vi "Impedance tube v0.3_cross_power.vi"() -> ()   [LabVIEW 2021]
uses:
  <vilib>/Analysis/2dsp.llb/Real FFT.vi
  <vilib>/express/express arith-compare/Formula/XNode/ExpressFormulaBlockNode.xnode
  <vilib>/Analysis/NI_AALPro.lvlib
panel:
  out "Transfer function 2":dbl[](graph)
  in  "dt":dbl=1.0 format="%0.2f"
  out "probe 1":dbl[](graph)
  out "Reflection coefficient":dbl[](graph)
  out "Absorption Coefficient":dbl[](graph)
  out "FFT {2}":cdb[](array[numeric])
  out "FFT {1}":cdb[](array[numeric])
  out "Transfer function":dbl[](graph)
  out "MIC 2":dynamicdata(graph)
  out "FFT2":dbl[](graph)
  in  "FFT size 2":i32=-1
  out "MIC 2":dbl
  out "FFT1":dbl[](graph)
  out "MIC 1":dynamicdata(graph)
  in  "FFT size":i32=-1
  out "MIC 1":dbl
  in  "stop (F)":bool
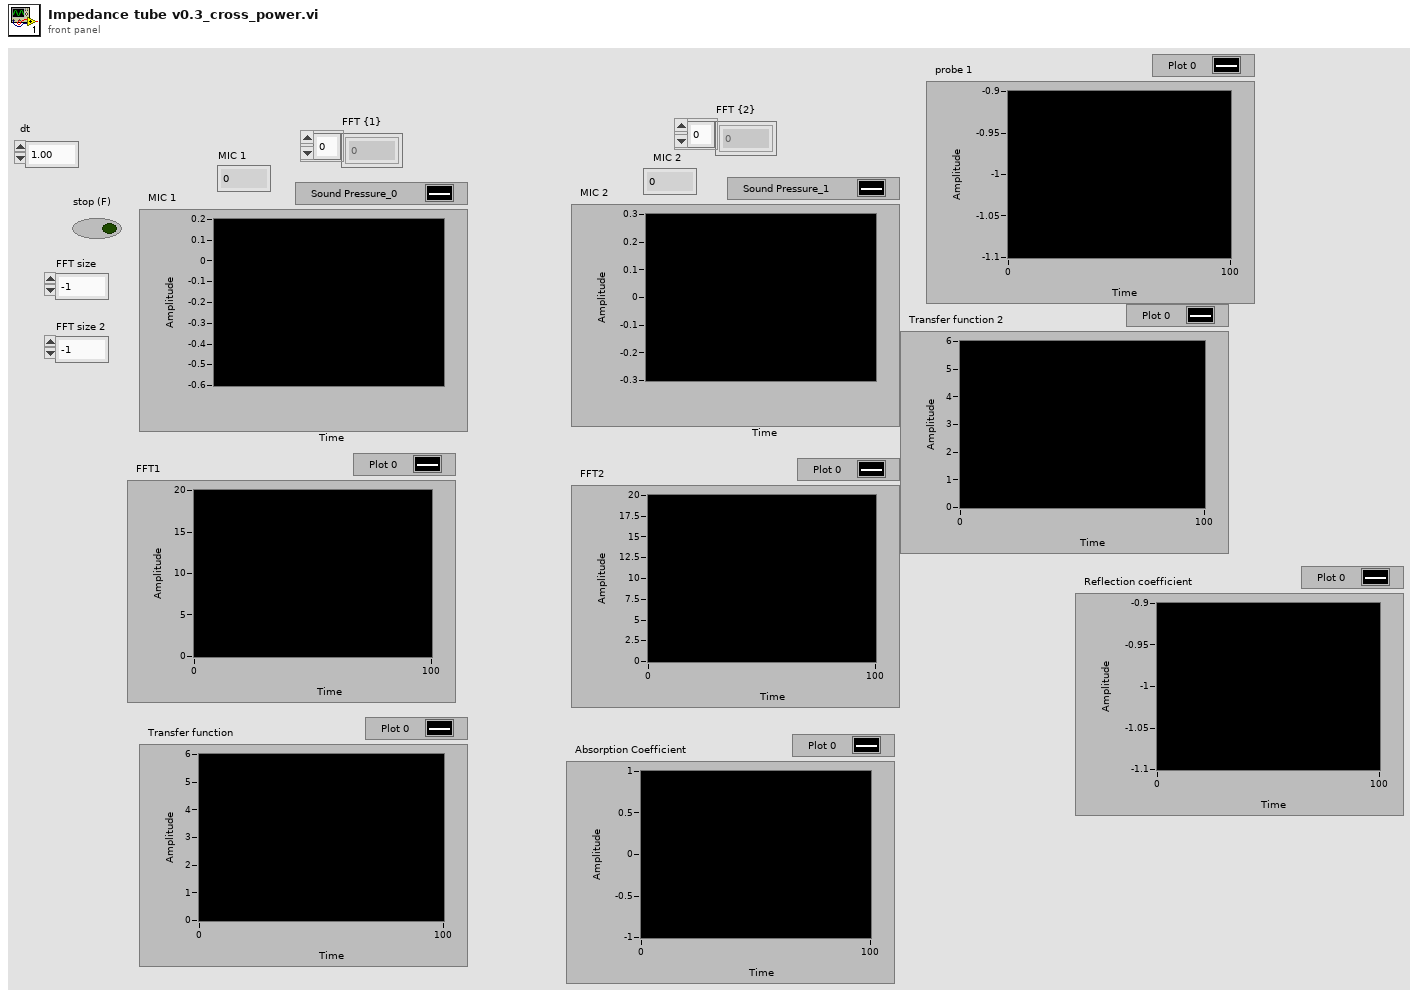
[diagram p1: front panel]
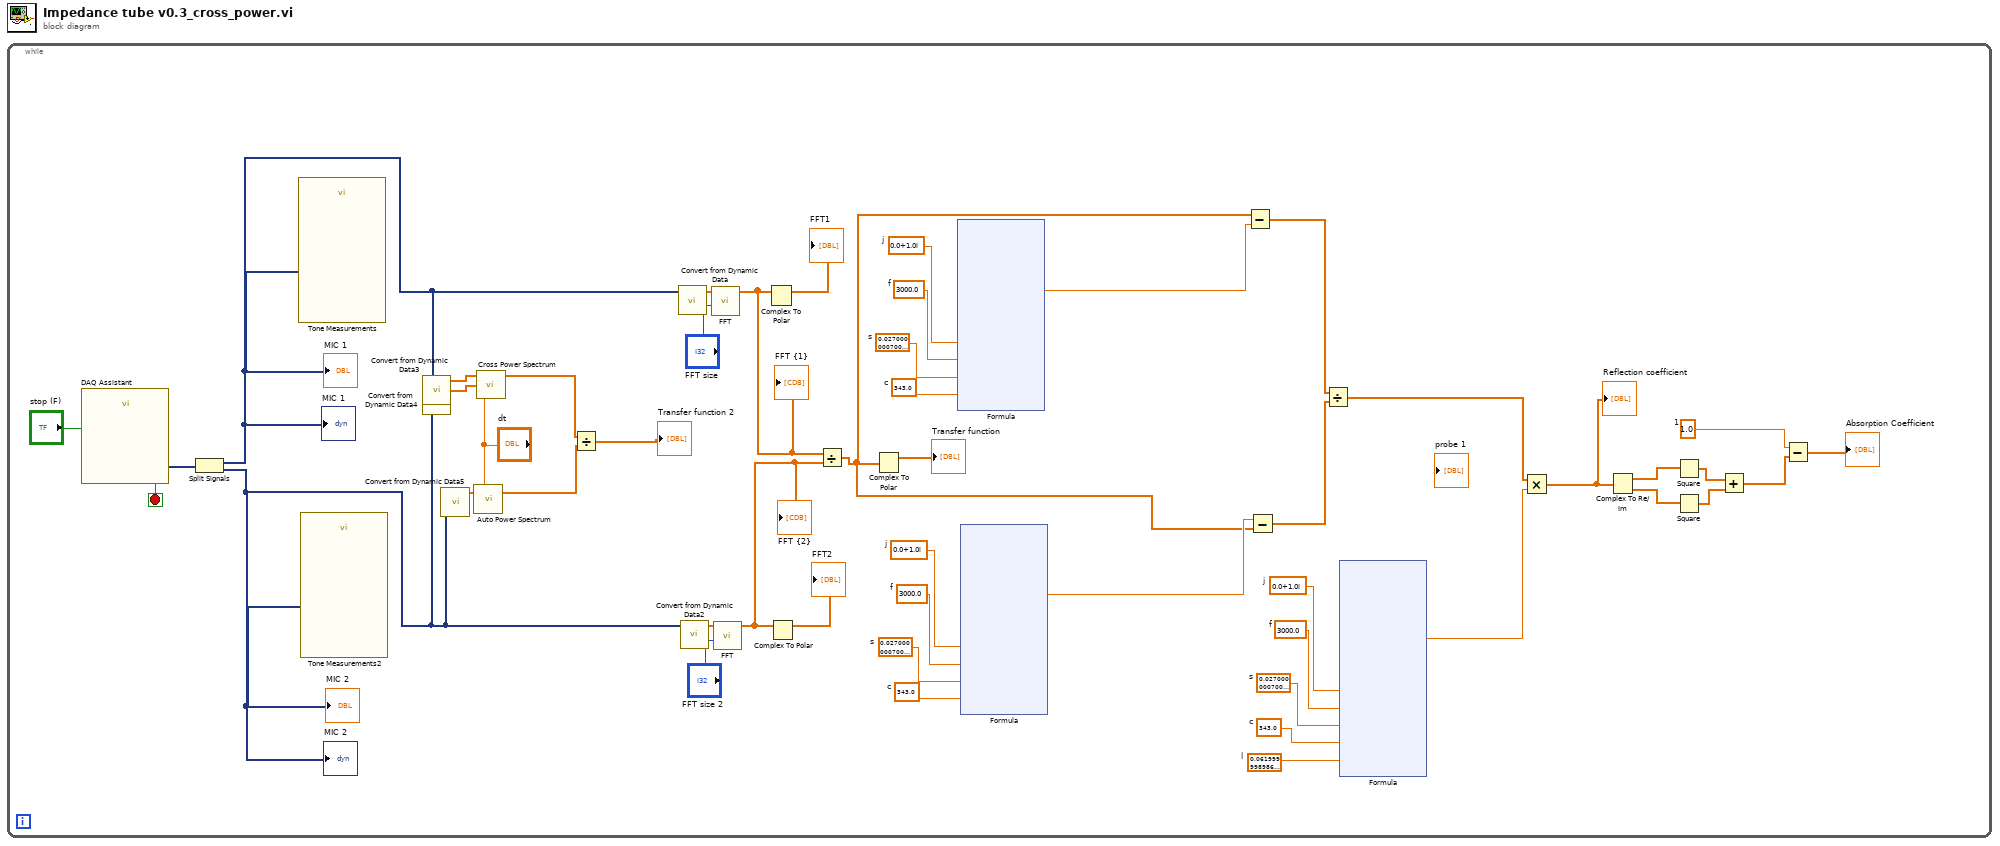
[diagram p0: block diagram]
diagram:
  n1 = while {
    stop <- w48 stop-if-true
    w17 = sgl 1.0  # 1
    w23 = sgl 0.062  # l
    w26 = sgl 3000.0  # f
    w25 = sgl 0.027  # s
    w24 = sgl 343.0  # c
    w27 = csg 0.0+1.0i  # j
    w31 = sgl 3000.0  # f
    w30 = sgl 0.027  # s
    w29 = sgl 343.0  # c
    w32 = csg 0.0+1.0i  # j
    w36 = sgl 3000.0  # f
    w35 = sgl 0.027  # s
    w34 = sgl 343.0  # c
    w37 = csg 0.0+1.0i  # j
    n2 = call "DAQ Assistant"("stop (F)"="stop (F)") -> ("data"=w44:dynamicdata, "stopped"=w48:bool)  [unwired: 15 in, 2 out]
    n3 = Split Signals(w44) -> (w9:dynamicdata, w6:dynamicdata)  [unwired: 2 in]
    "MIC 1" <- w9
    "MIC 1" <- w9
    "MIC 2" <- w6
    "MIC 2" <- w6
    n4 = call "Tone Measurements"("Signals"=w9) -> ()  [unwired: 8 in, 3 out]
    n5 = call "Tone Measurements2"("Signals"=w6) -> ()  [unwired: 8 in, 3 out]
    n6 = call "Convert from Dynamic Data3"("Dynamic Data Type"=w9) -> ("Array"=w8:dbl[])  [unwired: 3 in]
    n7 = call "Convert from Dynamic Data4"("Dynamic Data Type"=w6) -> ("Array"=w7:dbl[])  [unwired: 3 in]
    n8 = call "Convert from Dynamic Data5"("Dynamic Data Type"=w6) -> ("Array"=w5:dbl[])  [unwired: 3 in]
    n9 = call <vilib>:"Auto Power Spectrum.vi"("dt"="dt", "Signal (V)"=w5) -> ("Power Spectrum (V^2 rms)"=w2:dbl[])  [unwired: 1 out]
    n10 = call <vilib>:"Cross Power Spectrum.vi"("dt"="dt", "Signal Y (V)"=w7, "Signal X (V)"=w8) -> ("Cross Power XY Spectrum Mag (V^2rms)"=w3:dbl[])  [unwired: 2 out]
    n11 = Divide(x=w3, y=w2) -> (x/y=→"Transfer function 2":dbl[])
    n12 = call "Convert from Dynamic Data"("Dynamic Data Type"=w9) -> ("Array"=w46:dbl[])  [unwired: 3 in]
    n13 = call "Convert from Dynamic Data2"("Dynamic Data Type"=w6) -> ("Array"=w42:dbl[])  [unwired: 3 in]
    n14 = call-poly <vilib>:"FFT.vi"("FFT size"="FFT size", "X"=w46) -> ("FFT {X}"=w40:cdb[])  [unwired: 8 in, 1 out]
    "FFT {1}" <- w40
    n15 = call-poly <vilib>:"FFT.vi"("FFT size"="FFT size 2", "X"=w42) -> ("FFT {X}"=w39:cdb[])  [unwired: 8 in, 1 out]
    "FFT {2}" <- w39
    n16 = Complex To Polar(r * e^(i*theta)=w40) -> (r=→"FFT1":dbl[])  [unwired: 1 out]
    n17 = Complex To Polar(r * e^(i*theta)=w39) -> (r=→"FFT2":dbl[])  [unwired: 1 out]
    n18 = Divide(x=w40, y=w39) -> (x/y=w13:cdb[])
    n19 = Complex To Polar(r * e^(i*theta)=w13) -> (r=→"Transfer function":dbl[])  [unwired: 1 out]
    n20 = xnode "Formula"("j"=w37, "f"=w36, "s"=w35, "c"=w34) -> ("Result"=w33:dbl)  [unwired: 1 in, 1 out]
    n21 = xnode "Formula"("j"=w32, "f"=w31, "s"=w30, "c"=w29) -> ("Result"=w28:dbl)  [unwired: 1 in, 1 out]
    n22 = Subtract(x=w13, y=w33) -> (x-y=w12:cdb[])
    n23 = Subtract(x=w28, y=w13) -> (x-y=w11:cdb[])
    n24 = Divide(x=w12, y=w11) -> (x/y=w10:cdb[])
    n25 = xnode "Formula"("j"=w27, "f"=w26, "s"=w25, "c"=w24, "l"=w23) -> ("Result"=w22:dbl)  [unwired: 1 in, 1 out]
    n26 = Multiply(x=w10, y=w22) -> (x*y=w14:cdb[])
    "Reflection coefficient" <- w14
    n27 = Complex To Re/Im(x + iy=w14) -> (x=w21:dbl[], y=w20:dbl[])
    n28 = Square(x=w21) -> (x^2=w19:dbl[])
    n29 = Square(x=w20) -> (x^2=w18:dbl[])
    n30 = Add(x=w19, y=w18) -> (x+y=w16:dbl[])
    n31 = Subtract(x=w17, y=w16) -> (x-y=→"Absorption Coefficient":dbl[])
  }
